vi "dynamic Read Bytes.vi"(7 "pointer":u32, 8 "error in":errorcluster, 9 "dataLength":u32, 10 "targetAddress":u32, 11 "cycloneHandle":u32) -> (0 "error out":errorcluster, 3 "function return":bool, 5 "pointer out":u32)   [LabVIEW 2021, in "CycloneControlSDK.lvlib"]
doc: "extern \"C\" bool _cdecl dynamicReadBytes(uint32_t cycloneHandle, uint32_t targetAddress, uint32_t dataLength, void *pointer);"
uses:
  CycloneControlSDK.lvlib
  CycloneControlSDK_64.dll
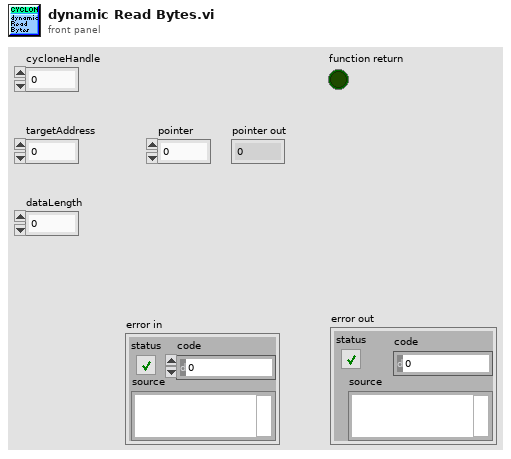
[diagram p1: front panel]
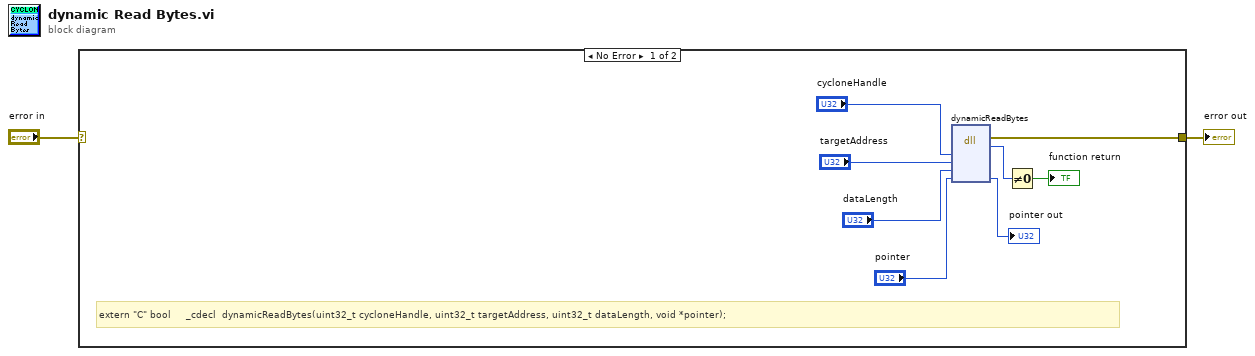
[diagram p0: block diagram]
diagram:
  n1 = case shown="No Error" "error in" {
    selector: "error in" -> [_ w11]
    tunnel: [w3 w11] -> w1
    frame No Error {
      # "extern \"C\" bool     _cdecl  dynamicReadBytes(uint32_t cycloneHandle, uint32_t targetAddress, uint32_t dataLength, void *pointer);"
      n2 = dll-call lib="C:/PEMicro/cyclone/cycloneControl/controlsdk/examples/labview2018/user.lib/CycloneControlSDK/CycloneControlSDK_64.dll" fn="dynamicReadBytes"("cycloneHandle"="cycloneHandle", "targetAddress"="targetAddress", "dataLength"="dataLength", "pointer"="pointer") -> (error out=w3:errorcluster, "return type"=w9:u8, "pointer"=→"pointer out":u32)  [unwired: 6 in, 1 out]
      n3 = Not Equal To 0?(x=w9) -> (x != 0?=→"function return":bool)
    }
    frame Error {
    }
  }
  "error out" <- w1
